vi "Test_Sinusoid.vi"() -> ()   [LabVIEW 2017]
panel:
  in  "stop (F)":bool
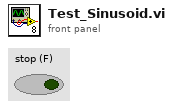
[diagram p1: front panel]
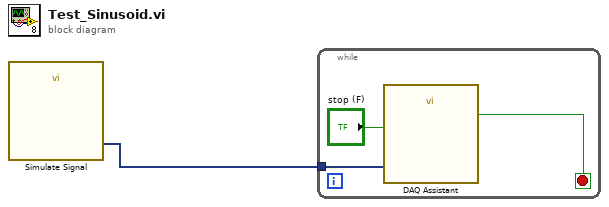
[diagram p0: block diagram]
diagram:
  n1 = call "Simulate Signal"() -> ("Sine"=w1:dynamicdata)  [unwired: 14 in, 1 out]
  n2 = while {
    tunnel: w1 -> [w2]
    stop <- w3 stop-if-true
    n3 = call "DAQ Assistant"("data"=w2, "stop (F)"="stop (F)") -> ("stopped"=w3:bool)  [unwired: 15 in, 2 out]
  }
